vi "Write Code.vi"(8 "error in (no error)":errorcluster, 10 "Code":dbl, 11 "SimpleEvent in":refnum<class "SimpleEvent.lvclass">) -> (0 "error out":errorcluster, 3 "SimpleEvent out":refnum<class "SimpleEvent.lvclass">)   [LabVIEW 2012, in "SimpleEvent.lvclass"]
uses:
  SimpleEvent.lvclass
  SimpleEvent.lvclass/SimpleEvent.ctl
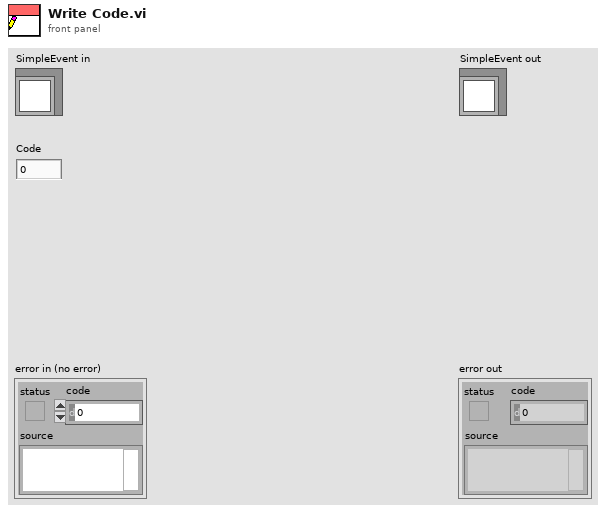
[diagram p1: front panel]
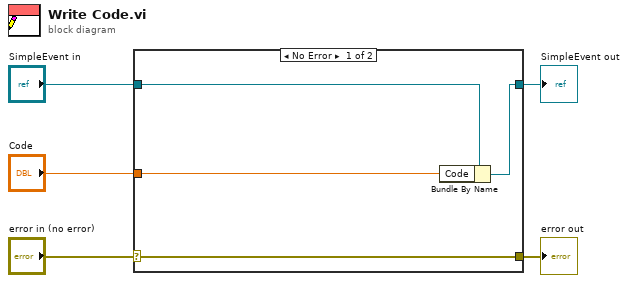
[diagram p0: block diagram]
diagram:
  n1 = case shown="No Error" "error in (no error)" {
    selector: "error in (no error)" -> [w9 w10]
    tunnel: [w9 w10] -> w4
    tunnel: [w7 w11] -> w2
    tunnel: "SimpleEvent in" -> [w8 w11]
    tunnel: "Code" -> [w6 _]
    frame No Error {
      n2 = Bundle By Name(cluster=w8, "Code"=w6) -> (w7:refnum<class "SimpleEvent.lvclass">)
    }
    frame Error {
    }
  }
  "error out" <- w4
  "SimpleEvent out" <- w2
